vi "Make.vi"(8 "error in (no error)":errorcluster, 9 "Item Refnum":refnum<vi>, 10 "Target":refnum<vi>, 11 "Coupled Message Rescripter":refnum<class "Coupled Message Rescripter.lvclass">) -> (0 "error out":errorcluster, 3 "Coupled Message Rescripter out":refnum<class "Coupled Message Rescripter.lvclass">)   [LabVIEW 2020, in "Message Rescripter.lvlib" / "Coupled Message Rescripter.lvclass"]
uses:
  Coupled Message Rescripter.lvclass
  MessageMakerProvider/_Message Maker/_Maker Classes/Message Scripter/Message Scripter.lvclass
  MessageMakerProvider/_Message Maker/_Maker Classes/Concrete Send Builder/Concrete Send Builder.lvclass
  Message Rescripter.lvlib
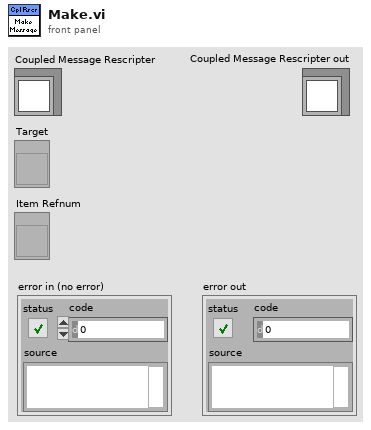
[diagram p1: front panel]
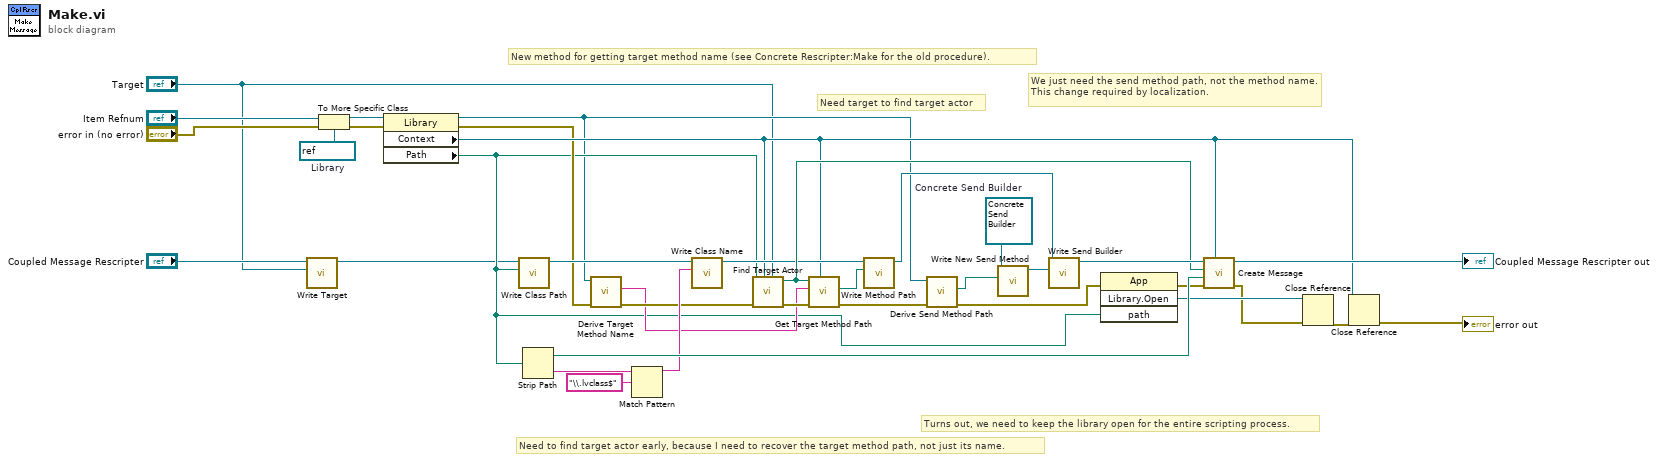
[diagram p0: block diagram]
diagram:
  w25 = refnum<vi> refnum  # Library
  w9 = refnum<class "Concrete Send Builder.lvclass"> refnum  # Concrete Send Builder
  # "Need target to find target actor"
  # "We just need the send method path, not the method name.  This change required by localization."
  # "New method for getting target method name (see Concrete Rescripter:Make for the old procedure)."
  # "Need to find target actor early, because I need to recover the target method path, not just its name."
  # "Turns out, we need to keep the library open for the entire scripting process."
  n1 = call "Write Target.vi"("Target"="Target", "Message Scripter in"="Coupled Message Rescripter") -> ("Message Scripter out"=w2:refnum<class "Coupled Message Rescripter.lvclass">)  [unwired: 9 in]
  n2 = To More Specific Class(target class=w25, reference="Item Refnum", error in="error in (no error)") -> (specific class reference=w27:refnum<vi>, error out=w26:errorcluster)
  n3 = property class="Library"(reference=w27, error in=w26) -> (reference out=w5:refnum<vi>, error out=w11:errorcluster, "Context"=w14:refnum<vi>, "Path"=w7:path)
  n4 = call "Write Class Path.vi"("Class Path"=w7, "Message Scripter in"=w2) -> ("Message Scripter out"=w36:refnum<class "Coupled Message Rescripter.lvclass">)  [unwired: 9 in]
  n5 = Strip Path(path=w7) -> (stripped path=w34:path, name=w20:string)
  n6 = call "Derive Target Method Name.vi"("error in (no error)"=w11, "Library"=w5) -> ("error out"=w12:errorcluster, "Likely Target Method"=w10:string)  [unwired: 8 in]
  n7 = Match Pattern(string=w20, regular expression="\\.lvclass$") -> (before substring=w13:string)  [unwired: 1 in, 3 out]
  n8 = call "Write Class Name.vi"("Class Name"=w13, "Message Scripter in"=w36) -> ("Message Scripter out"=w16:refnum<class "Coupled Message Rescripter.lvclass">)  [unwired: 9 in]
  n9 = call "Find Target Actor.vi"("Target"="Target", "App Inst"=w14, "error in (no error)"=w12, "Message Path"=w7) -> ("error out"=w17:errorcluster, "Targeted Actor"=w18:path)  [unwired: 6 in]
  n10 = call "Get Target Method Path.vi"("App Inst"=w14, "error in (no error)"=w17, "Target Method"=w10, "Target Actor Path"=w18) -> ("error out"=w6:errorcluster, "Target Method Path"=w15:path)  [unwired: 6 in]
  n11 = call "Write Method Path.vi"("Method Path"=w15, "Message Scripter in"=w16) -> ("Message Scripter out"=w8:refnum<class "Coupled Message Rescripter.lvclass">)  [unwired: 9 in]
  n12 = call "Derive Send Method Path.vi"("error in (no error)"=w6, "Library"=w5) -> ("error out"=w4:errorcluster, "Send VI Path"=w31:path)  [unwired: 7 in, 1 out]
  n13 = call "Write New Send Method.vi"("New Send Method"=w31, "Concrete Send Builder in"=w9) -> ("Concrete Send Builder out"=w33:refnum<class "Concrete Send Builder.lvclass">)  [unwired: 9 in]
  n14 = call "Write Send Builder.vi"("Message Maker.lvlib:Send Builder.lvclass"=w33, "Message Scripter in"=w8) -> ("Message Scripter out"=w32:refnum<class "Coupled Message Rescripter.lvclass">)  [unwired: 9 in]
  n15 = invoke class="App" method="Library.Open"(error in=w4, "path"=w7) -> (error out=w19:errorcluster, "Open Library"=w30:refnum<vi>)  [unwired: 2 in, 2 out]
  n16 = call "Create Message.vi"("AppInst"=w14, "error in (no error)"=w19, "Destination Path"=w34, "Actor class path"=w18, "Message Maker in"=w32) -> ("error out"=w29:errorcluster, "Message Maker out"=→"Coupled Message Rescripter out":refnum<class "Coupled Message Rescripter.lvclass">)  [unwired: 5 in]
  n17 = Close Reference(reference=w30, error in (no error)=w29) -> (error out=w28:errorcluster)
  n18 = Close Reference(reference=w14, error in (no error)=w28) -> (error out=→"error out":errorcluster)
